vi "Actor Core.vi"(8 "error in":errorcluster, 11 "FunctionGenerator in":refnum<class "FunctionGenerator.lvclass">) -> (0 "error out":errorcluster, 3 "Actor out":refnum<class "Actor.lvclass">)   [LabVIEW 2019, in "FunctionGenerator.lvlib" / "FunctionGenerator.lvclass"]
doc: "The instrument actor core is only here to distribute panel resolution settings to children classes."
uses:
  Library/FunctionGenerator.lvclass
  builds/Engine/Actor Framework.lvlibp/1abvi3w/vi.lib/ActorFramework/Actor/Actor.lvclass
  Custom Controls/WaveformSettings.ctl
  Custom Controls/WaveformMode.ctl
  FunctionGenerator Messages/Configure Channel Msg/Configure Channel Msg.lvclass/Configure Channel Msg.ctl
  FunctionGenerator Messages/Select Channel Msg/Select Channel Msg.lvclass/Select Channel Msg.ctl
  builds/Engine/Actor Framework.lvlibp/1abvi3w/vi.lib/ActorFramework/Message Enqueuer/Enqueue.vi
  FunctionGenerator Messages/Configure Channel Msg/Configure Channel Msg.lvclass
  FunctionGenerator Messages/Select Channel Msg/Select Channel Msg.lvclass
  builds/Instruments/Instruments.lvlibp/Library/Instruments.lvclass
  C:/Users/Public/Documents/Development/builds/Instruments/Instruments.lvlibp/Library/Instruments.lvclass
panel:
  out "OutputStat":bool
  in  "Active Device":u16(ring)
  in  "Settings":T1 {"Fall Time" format="%#_g s"; "Rise Time" format="%#_g s"; "Pulse Width" format="%#_g s"; "Symmetry" format="%#_g %"; "Phase" format="%#_g °"; "Offset" format="%#_g V"; "Amplitude" format="%#_g V"; "Frequency" format="%^2.0g"}
  in  "Channel":u16(ring)
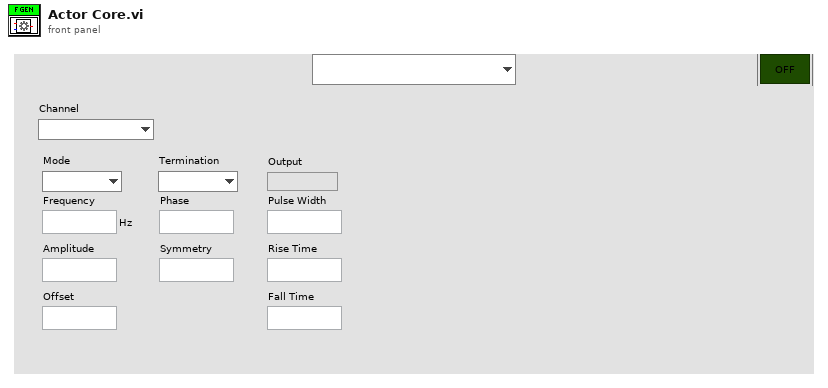
[diagram p1: front panel]
types:
  T1 = typedef "FunctionGenerator.lvlib/FunctionGenerator.lvclass/WaveformSettings.ctl" = cluster{"Frequency":dbl, "Amplitude":dbl, "Offset":dbl, "Phase":dbl, "Symmetry":dbl, "Pulse Width":dbl, "Rise Time":dbl, "Fall Time":dbl, "Mode":T2, "Termination":enum16{"50_Ohm", "High_Z"}, "Output":bool}
  T2 = typedef "FunctionGenerator.lvlib/FunctionGenerator.lvclass/WaveformMode.ctl" = enum16{"Sine", "Square", "Ramp", "Pulse", "Arbitrary", "Triangle", "Noise", "DC"}
  T3 = cluster{"Pnl Actor":refnum<event-registration>, "Event Registration Refnum":refnum<event-registration>}
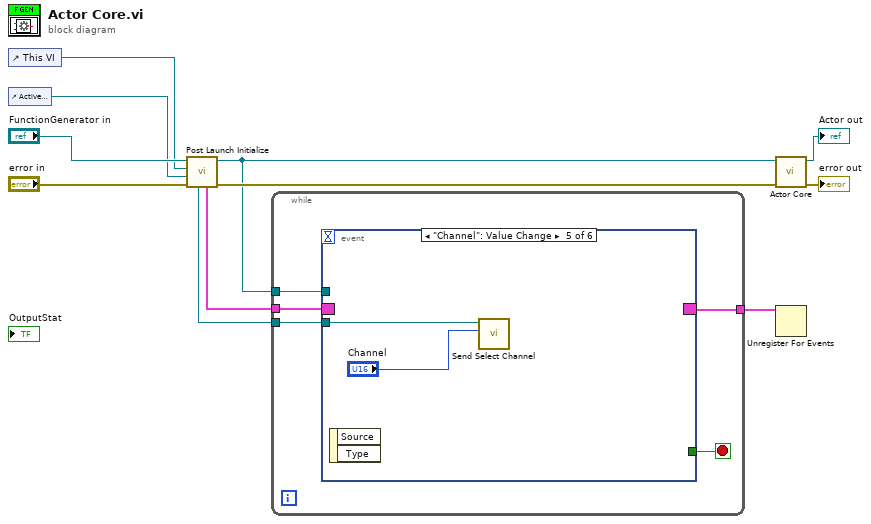
[diagram p0: block diagram]
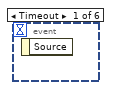
[diagram p2: hidden frame]
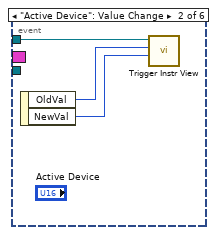
[diagram p3: hidden frame]
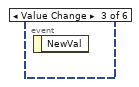
[diagram p4: hidden frame]
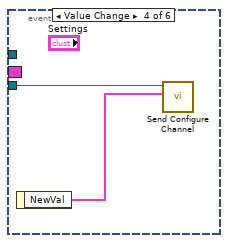
[diagram p5: hidden frame]
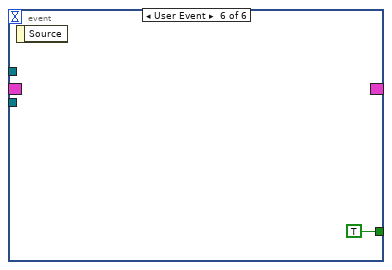
[diagram p6: hidden frame]
diagram:
  n1 = control-ref of="This VI"() -> (w6:refnum<vi>)
  n2 = control-ref of="Active Device"() -> (w5:refnum<vi>)
  n3 = call "Post Launch Initialize.vi"("error in"="error in", "Active Device"=w5, "GUI Reference"=w6, "Instruments in"="FunctionGenerator in") -> ("error out"=w8:errorcluster, "Instruments out"=w2:refnum<class "FunctionGenerator.lvclass">, "Registered Events"=w4:T3, "Self Enqueuer"=w3:refnum<class "Message Enqueuer.lvclass">)  [unwired: 4 in]
  n4 = while {
    tunnel: w4 -> [w16]
    tunnel: w3 -> [w14]
    tunnel: w2 -> [w15]
    tunnel: [w12] -> w1
    stop <- w13 stop-if-true
    n5 = event shown="[4] \"Channel\": Value Change" {
      selector: w16 -> [_ _ _ _ _ _]
      dyn-events: [_ _ _ _ _ _] -> w12
      timeout: _ -> [_ _ _ _ _ _]
      tunnel: w15 -> [_ w19 _ _ _ _]
      tunnel: w14 -> [_ _ _ w21 w23 _]
      tunnel: [_ _ _ _ _ TRUE] -> w13
      event Timeout {
        n6 = event-data() -> ()  [unwired: 1 in, 1 out]
      }
      event "Active Device": Value Change {
        n7 = event-data() -> ("OldVal"=w18:u16, "NewVal"=w17:u16)  [unwired: 1 in]
        n8 = call "Trigger Instr View.vi"("New Value"=w17, "Old Value"=w18, "Instruments in"=w19) -> ()  [unwired: 7 in, 2 out]
      }
      event Value Change {
        n9 = event-data() -> ()  [unwired: 1 in, 1 out]
      }
      event Value Change {
        n10 = event-data() -> ("NewVal"=w20:T1)  [unwired: 1 in]
        n11 = call "Send Configure Channel.vi"("Settings"=w20, "Message Enqueuer"=w21) -> ()  [unwired: 8 in, 2 out]
      }
      event "Channel": Value Change {
        n12 = event-data() -> ()  [unwired: 1 in, 2 out]
        n13 = call "Send Select Channel.vi"("Active Channel"="Channel", "Message Enqueuer"=w23) -> ()  [unwired: 8 in, 2 out]
      }
      event User Event {
        n14 = event-data() -> ()  [unwired: 1 in, 1 out]
      }
    }
  }
  n15 = call-parent "Actor Core.vi"("error in"=w8, "Instruments in"=w2) -> ("error out"=→"error out":errorcluster, "Actor out"=→"Actor out":refnum<class "Actor.lvclass">)  [unwired: 8 in]
  n16 = Unregister For Events(event registration refnum=w1) -> ()  [unwired: 1 in, 1 out]
